vi "MGI SZL UnZip To Directory.vi"(8 "Error In":errorcluster, 9 "Target Directory":path, 10 "Preview Only? (F)":bool, 11 "Zip File":path=path "D:/temp/Top.zip") -> (0 "Error Out":errorcluster, 2 "Preview[]":string[](array[string]), 3 "Uzipped File[]":path[](array[path]))   [LabVIEW 2020]
doc: "Unzips the contents of zip file to the target directory. If Preview only? is true, this VI doesn't unzip the contents and just returns a preview of the list of files.\n\nThis VI relies on the Sharp Zip Library which is a .NET assembly written in C# by Mike Krueger. It is licenced under the GPL with a special exception permitting independent modules to link to the library regardless of the license terms of the independent module. \n\nMore information about the library and its license is available from:\nhttp://www.icsharpcode.net/opensource/sharpziplib/\n\nAuthored by Matthew G. Harrison\nsupport@mooregoodideas.com\nwww.mooregoodideas.com\n\nCopyright (c) 2010, Moore Good Ideas, Inc.\n\nAll rights reserved.\n\nRedistribution and use in source and binary forms, with or without modification, are permitted provided that the following conditions are met:\n\n * Redistributions of source code must retain the above copyright notice, this list of conditions and the following disclaimer.\n * Redistributions in binary form must reproduce the above copyright notice, this list of conditions and the following disclaimer in the documentation and/or other materials provided with the distribution.\n * Neither the name of Moore Good Ideas, Inc. nor the names of its contributors may be used to endorse or promote products derived from this software without specific prior written permission.\n\nTHIS SOFTWARE IS PROVIDED BY THE COPYRIGHT HOLDERS AND CONTRIBUTORS \"AS IS\" AND ANY EXPRESS OR IMPLIED WARRANTIES, INCLUDING, BUT NOT LIMITED TO, THE IMPLIED WARRANTIES OF MERCHANTABILITY AND FITNESS FOR A PARTICULAR PURPOSE ARE DISCLAIMED. IN NO EVENT SHALL THE COPYRIGHT OWNER OR CONTRIBUTORS BE LIABLE FOR ANY DIRECT, INDIRECT, INCIDENTAL, SPECIAL, EXEMPLARY, OR CONSEQUENTIAL DAMAGES (INCLUDING, BUT NOT LIMITED TO, PROCUREMENT OF SUBSTITUTE GOODS OR SERVICES; LOSS OF USE, DATA, OR PROFITS; OR BUSINESS INTERRUPTION) HOWEVER CAUSED AND ON ANY THEORY OF LIABILITY, WHETHER IN CONTRACT, STRICT LIABILITY, OR TORT (INCLUDING NEGLIGENCE OR OTHERWISE) ARISING IN ANY WAY OUT OF THE USE OF THIS SOFTWARE, EVEN IF ADVISED OF THE POSSIBILITY OF SUCH DAMAGE."
uses:
  <userlib>/_MGI/File/MGI Create Directory Chain Behavior Enum.ctl
  C:/Program Files/National Instruments/LabVIEW 2020/user.lib/_MGI/File/Zip/Support Files/ICSharpCode.SharpZipLib.dll
  Support Files/ICSharpCode.SharpZipLib.dll
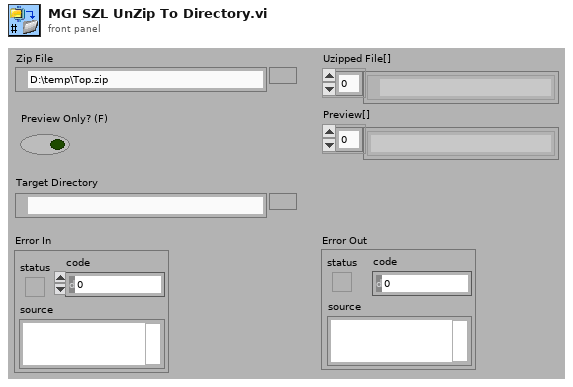
[diagram p1: front panel]
types:
  T1 = typedef "MGI Create Directory Chain Behavior Enum.ctl" = enum16{"Auto Detect", "Path Contains a File", "Path Does Not Contain a File"}
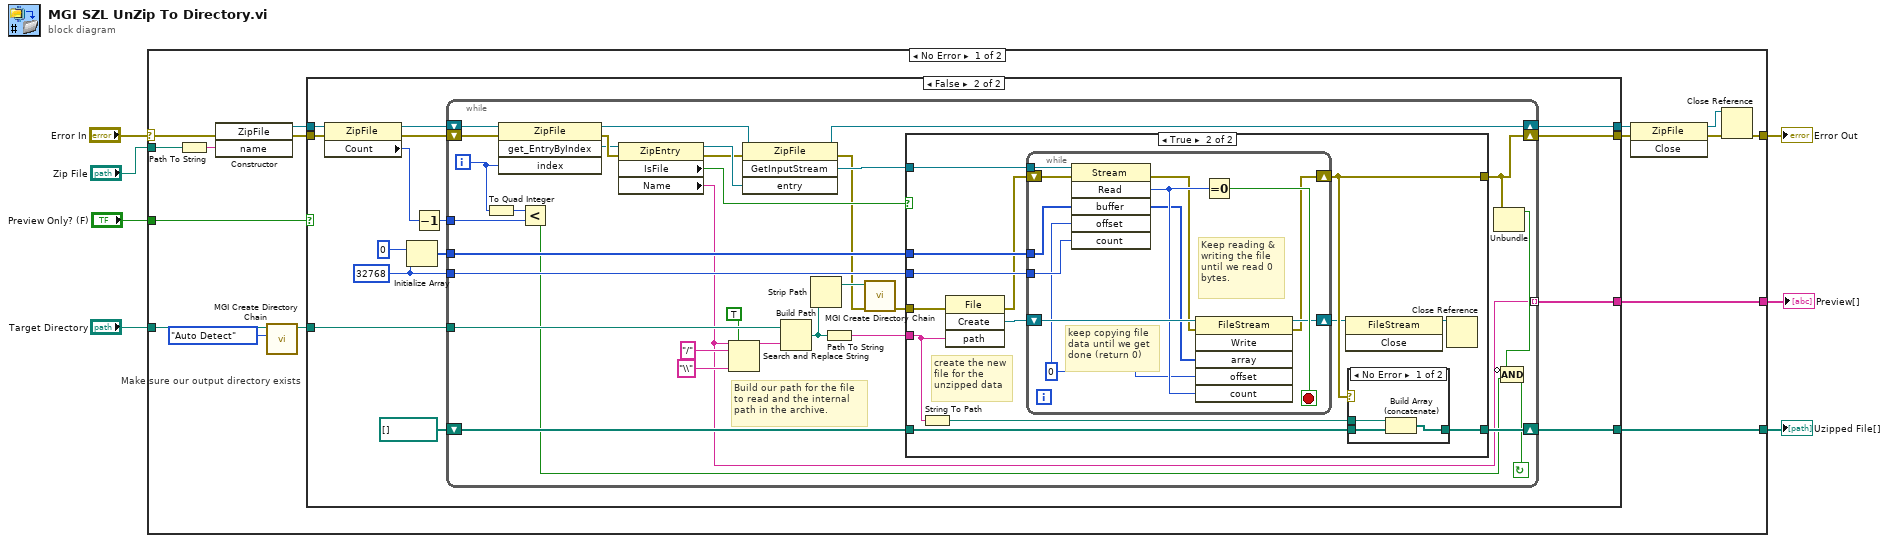
[diagram p0: block diagram]
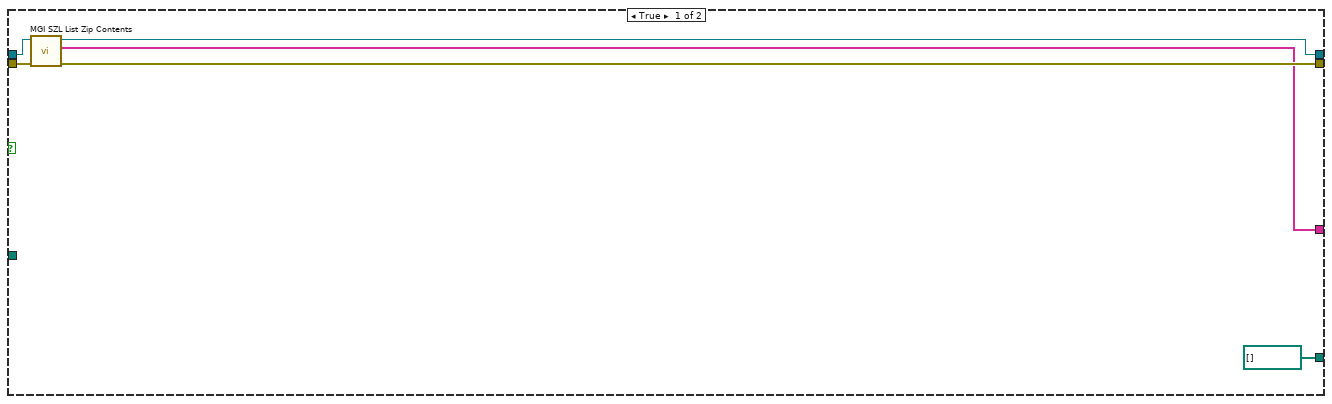
[diagram p2: hidden frame]
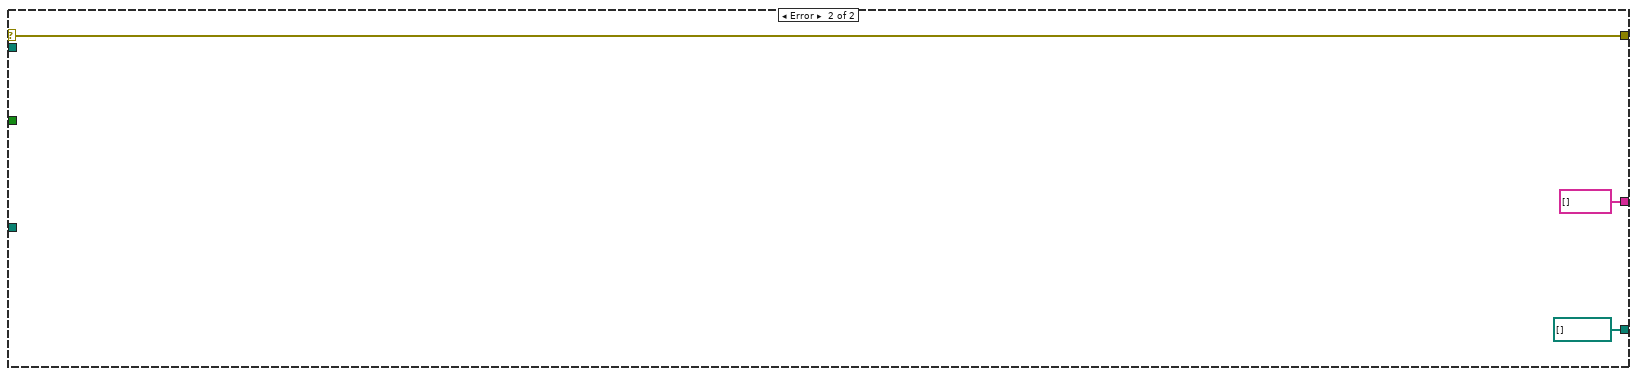
[diagram p5: hidden frame]
diagram:
  n1 = case shown="No Error" "Error In" {
    selector: "Error In" -> [w12 w110]
    tunnel: [w22 w110] -> w7
    tunnel: "Zip File" -> [w17 _]
    tunnel: "Target Directory" -> [w9 _]
    tunnel: [w16 path[] []] -> w4
    tunnel: "Preview Only? (F)" -> [w14 _]
    tunnel: [w13 string[] [] ("file names")] -> w2
    frame No Error {
      n2 = Path To String(path=w17) -> (string=w18:string)
      n3 = constructor class="ZipFile"(error in=w12, "name"=w18) -> (reference out=w11:refnum<k24>, error out=w15:errorcluster)  [unwired: 2 in, 2 out]
      n4 = call <userlib>:"MGI Create Directory Chain.vi"("File Presence (Auto Detect)"=MGI_Create_Directory_Chain_Behavior_Enum."Auto Detect", "Path"=w9) -> ("Duplicate Path"=w8:path)  [unwired: 8 in, 1 out]
      n5 = case shown="False" w14 {
        tunnel: [w27 w44] -> w20
        tunnel: [w26 w43] -> w19
        tunnel: w8 -> [_ w39]
        tunnel: [path[] [] w36] -> w16
        tunnel: w15 -> [w28 w35]
        tunnel: w11 -> [w29 w34]
        tunnel: [w24 w30] -> w13
        frame True {
          n6 = call <userlib>:"MGI SZL List Zip Contents.vi"("Error In"=w28, "Zip File"=w29) -> ("Error Out"=w27:errorcluster, "File Name[]"=w24:string[], "Zip File Out"=w26:refnum<k24>)  [unwired: 1 in, 6 out]
        }
        frame False {
          w40 = 32768 ("dimension size")
          # "Make sure our output directory exists"
          n7 = property class="ZipFile"(reference=w34, error in=w35) -> (reference out=w37:refnum<k24>, error out=w38:errorcluster, "Count"=w32:i64)
          n8 = Initialize Array(u8 0, w40) -> (w41:u8[])
          n9 = Decrement(x=w32) -> (x-1=w31:i64)
          n10 = while {
            shift-right: [w66] -> w43
            shift-left: w37 -> [w70]
            shift-right: [w52] -> w44
            shift-left: w38 -> [w76]
            tunnel: w41 -> [w73]
            tunnel: w40 -> [w72]
            tunnel: w39 -> [w71]
            shift-right: [w56] -> w36
            shift-left: path[] [] -> [w57]
            tunnel: w31 -> [w54]
            tunnel: [w48] -> w30 mode=indexing
            i -> [w55]
            stop <- w50 continue-if-true
            # "Build our path for the file\nto read and the internal\npath in the archive."
            n11 = To Quad Integer(1:w55) -> (0:w53:i64)
            n12 = invoke class="ZipFile" method="get_EntryByIndex"(reference=w70, error in=w76, "index"=w55) -> (reference out=w67:refnum<k24>, error out=w75:errorcluster, "get_EntryByIndex"=w74:refnum<k24>)  [unwired: 1 in, 1 out]
            n13 = Less?(x=w53, y=w54) -> (x < y?=w49:bool)
            n14 = property class="ZipEntry"(reference=w74, error in=w75) -> (reference out=w65:refnum<k24>, error out=w63:errorcluster, "IsFile"=w68:bool, "Name"=w48:string)
            n15 = Search and Replace String(replace all?=TRUE ("replace all? (F)"), input string=w48, search string="/", replace string="\\" ("replace string (\"\")")) -> (result string=w59:string)  [unwired: 1 in, 6 out]
            n16 = invoke class="ZipFile" method="GetInputStream"(reference=w67, error in=w63, "entry"=w65) -> (reference out=w66:refnum<k24>, error out=w46:errorcluster, "GetInputStream"=w64:refnum<k24>)  [unwired: 1 in, 1 out]
            n17 = Build Path(base path=w71, name or relative path=w59) -> (appended path=w58:path)
            n18 = Strip Path(path=w58) -> (stripped path=w47:path)  [unwired: 1 out]
            n19 = Path To String(path=w58) -> (string=w69:string)
            n20 = call <userlib>:"MGI Create Directory Chain.vi"("Error In"=w46, "Path"=w47) -> ("Error Out"=w45:errorcluster)  [unwired: 8 in, 1 out]
            n21 = case shown="True" w68 {
              tunnel: w64 -> [_ w91]
              tunnel: w73 -> [_ w90]
              tunnel: w72 -> [_ w88]
              tunnel: [w78 w85] -> w52
              tunnel: w69 -> [_ w82]
              tunnel: w45 -> [w78 w86]
              tunnel: w57 -> [w77 w84]
              tunnel: [w77 w83] -> w56
              frame False {
              }
              frame True {
                # "create the new\nfile for the \nunzipped data"
                n22 = String To Path(string=w82) -> (path=w81:path)
                n23 = invoke class="File" method="Create"(error in=w86, "path"=w82) -> (error out=w87:errorcluster, "Create"=w89:refnum<k24>)  [unwired: 2 in, 2 out]
                n24 = while {
                  tunnel: w91 -> [w107]
                  tunnel: w90 -> [w97]
                  tunnel: w88 -> [w105]
                  shift-right: [w98] -> w85
                  shift-left: w87 -> [w104]
                  shift-right: [w100] -> w80
                  shift-left: w89 -> [w106]
                  stop <- w102 stop-if-true
                  w101 = 0 ("offset")
                  # "Keep reading &\nwriting the file \nuntil we read 0\nbytes."
                  # "keep copying file\ndata until we get\ndone (return 0)"
                  n25 = invoke class="Stream" method="Read"(reference=w107, error in=w104, "buffer"=w97, "offset"=w101, "count"=w105) -> (error out=w99:errorcluster, "Read"=w103:i32, "buffer"=w96:u8[])  [unwired: 1 in, 3 out]
                  n26 = invoke class="FileStream" method="Write"(reference=w106, error in=w99, "array"=w96, "offset"=w101, "count"=w103) -> (reference out=w100:refnum<k24>, error out=w98:errorcluster)  [unwired: 1 in, 4 out]
                  n27 = Equal To 0?(x=w103) -> (x = 0?=w102:bool)
                }
                n28 = invoke class="FileStream" method="Close"(reference=w80) -> (reference out=w79:refnum<k24>)  [unwired: 2 in, 2 out]
                n29 = case shown="No Error" w85 {
                  tunnel: w84 -> [w94 w95]
                  tunnel: w81 -> [w93 _]
                  tunnel: [w92 w95] -> w83
                  frame No Error {
                    n30 = Build Array (concatenate)(w93, w94) -> (w92:path[])
                  }
                  frame Error {
                  }
                }
                n31 = Close Reference(reference=w79) -> ()  [unwired: 1 in, 1 out]
              }
            }
            n32 = Unbundle(w52) -> ("status"=w51:bool)  [unwired: 2 out]
            n33 = Compound Arithmetic op=AND(invert w51, w49) -> (w50:bool)
          }
        }
      }
      n34 = invoke class="ZipFile" method="Close"(reference=w19, error in=w20) -> (reference out=w21:refnum<k24>, error out=w23:errorcluster)  [unwired: 1 in, 1 out]
      n35 = Close Reference(reference=w21, error in (no error)=w23) -> (error out=w22:errorcluster)
    }
    frame Error {
    }
  }
  "Preview[]" <- w2
  "Error Out" <- w7
  "Uzipped File[]" <- w4
